vi "DisplayData.vi"(8 "error in (no error)":errorcluster caption="错误输入（无错误）", 11 "DigitalDisplay 输入":refnum<class "DigitalDisplay.lvclass">) -> (0 "error out":errorcluster caption="错误输出", 3 "DigitalDisplay 输出":refnum<class "DigitalDisplay.lvclass">)   [LabVIEW 2018, in "DataDisplay.lvlib" / "DigitalDisplay.lvclass"]
uses:
  DigitalDisplay.lvclass
  DigitalDisplay.lvclass/DigitalDisplay.ctl
  DataDisplay.lvlib
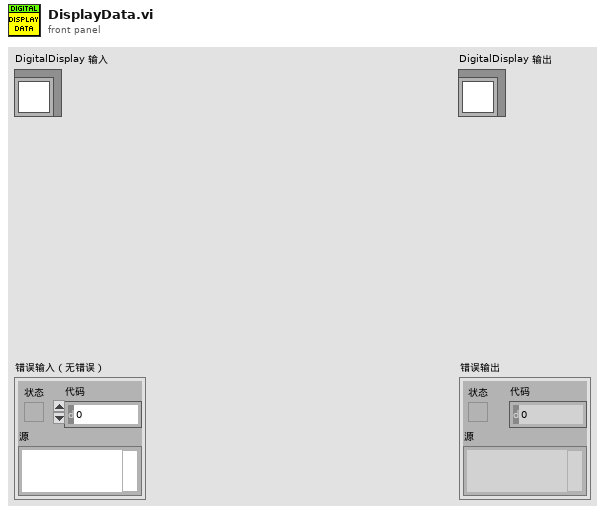
[diagram p1: front panel]
types:
  T1 = typedef "DataDisplay.lvlib/DD_DataStream.ctl" = cluster{"Data":dbl[]}[]
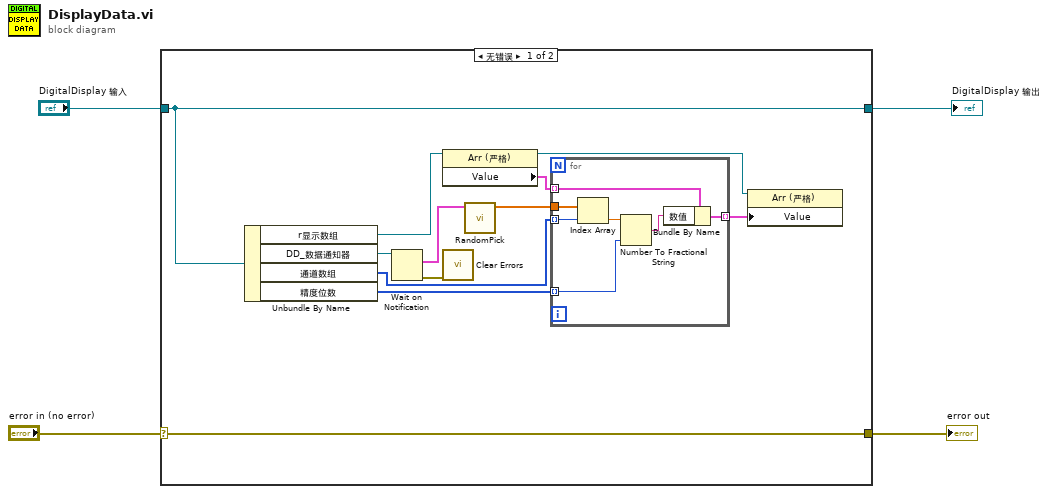
[diagram p0: block diagram]
diagram:
  n1 = case shown="无错误" "error in (no error)" {
    selector: "error in (no error)" -> [w16 w25]
    tunnel: [w16 w25] -> w3
    tunnel: [w14 w24] -> w1
    tunnel: "DigitalDisplay 输入" -> [w14 w24]
    frame No Error {
      n2 = Unbundle By Name(w14) -> ("r显示数组"=w9:refnum<vi>, "DD_数据通知器"=w10:refnum<notifier>, "通道数组"=w13:i32[], "精度位数"=w12:i32[])
      n3 = Wait on Notification(notifier=w10) -> (notification=w6:T1, error out=w15:errorcluster)  [unwired: 3 in, 2 out]
      n4 = property class="Arr (严格)"(reference=w9) -> (reference out=w8:refnum<vi>, "Value"=w11:cluster{"通道选择":u16, "数值":string}[])  [unwired: 1 in, 1 out]
      n5 = call <vilib>:"Clear Errors.vi"("error in (no error)"=w15) -> ()  [unwired: 5 in, 2 out]
      n6 = call "RandomPick.vi"("DataIn"=w6) -> ("DataOut"=w5:dbl[])  [unwired: 10 in]
      n7 = for {
        tunnel: w13 -> [w19] mode=indexing
        tunnel: w5 -> [w23]
        tunnel: [w22] -> w7 mode=indexing
        tunnel: w12 -> [w20] mode=indexing
        tunnel: w11 -> [w18] mode=indexing
        n8 = Index Array(array=w23, index=w19) -> (element=w17:dbl)
        n9 = Number To Fractional String(number=w17, precision (6)=w20) -> (F-format string=w21:string)  [unwired: 2 in]
        n10 = Bundle By Name(cluster=w18, "数值"=w21) -> (w22:cluster{"通道选择":u16, "数值":string})
      }
      n11 = property class="Arr (严格)"(reference=w8, "Value"=w7) -> ()  [unwired: 1 in, 2 out]
    }
    frame Error {
    }
  }
  "error out" <- w3
  "DigitalDisplay 输出" <- w1
